vi "1.HelloWorld.vi"() -> ()   [LabVIEW 2011]
panel:
  out "WriteSF Error":errorcluster
  out "OpenSF Error":errorcluster
  in  "Steering":u8(slide)=128 scale=0.0..255.0
  in  "Motor Speed":u8(slide)=128 scale=0.0..255.0
  in  "Destination Id":u8=7
  # "Left"
  # "Right"
  # "Full Forward"
  # "Full Rverse"
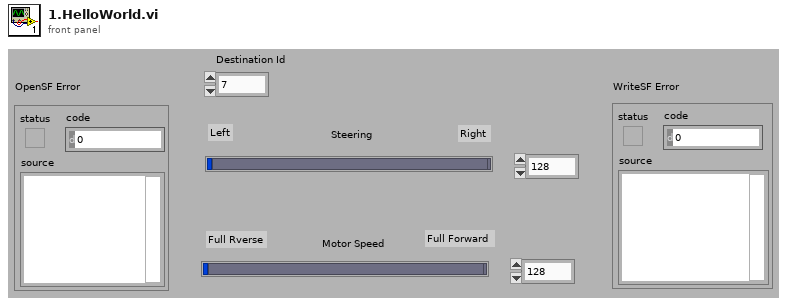
[diagram p1: front panel]
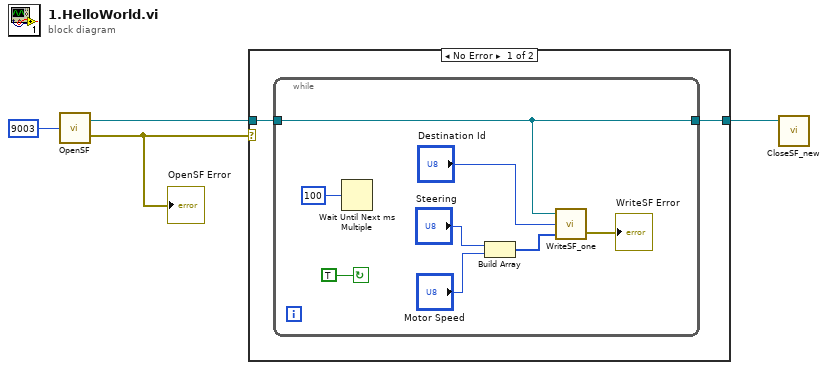
[diagram p0: block diagram]
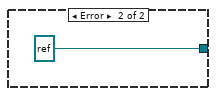
[diagram p2: hidden frame]
diagram:
  n1 = call "OpenSF.vi"("Port number"=u16 9003 ("Port number\nactuators")) -> ("connection ID"=w2:refnum<k5>, "Error out"=w3:errorcluster)
  "OpenSF Error" <- w3
  n2 = case shown="No Error" w3 {
    tunnel: w2 -> [w6 _]
    tunnel: [w5 refnum<k5> refnum ("connection ID")] -> w1
    frame No Error {
      n3 = while {
        tunnel: w6 -> [w10]
        tunnel: [w10] -> w5
        stop <- TRUE continue-if-true
        n4 = Wait Until Next ms Multiple(millisecond multiple=u32 100) -> ()  [unwired: 1 out]
        n5 = Build Array("Steering", "Motor Speed") -> (w8:u8[])
        n6 = call "WriteSF_one.vi"("payload"=w8, "destination ID"="Destination Id", "connection ID in"=w10) -> ("error out"=→"WriteSF Error":errorcluster)  [unwired: 1 out]
      }
    }
    frame Error {
    }
  }
  n7 = call "CloseSF_new.vi"("connection ID"=w1) -> ()  [unwired: 2 in]
